vi "Autofocus.vi"(0 "controller in":refnum<k24>, 1 "AbortAutoFocus":bool, 2 "ImageIn":T2, 5 "SafeMaxZ":dbl=86.0 format="%#_13g", 7 "InitialStepSize":dbl=0.1, 9 "Tolerance":dbl=0.005 format="%#_13g", 11 "error in (no error)":errorcluster, 12 "SessionIn":T1) -> (4 "controller out":refnum<k24>, 6 "Image":T2(plugin-control), 8 "N_iterations":dbl, 10 "BestZvalue":dbl, 14 "Session Out":T1, 15 "error out":errorcluster)   [LabVIEW 2021, in "Test VIs.lvclass"]
uses:
  Test VIs/Test VIs.lvclass
  C:/Program Files (x86)/Aerotech/A3200/LabVIEW/2010/Bin/Aerotech.A3200.dll
  Program Files (x86)/Aerotech/A3200/LabVIEW/2010/Bin/Aerotech.A3200.dll
  <vilib>/vision/Image Controls.llb/IMAQ Image.ctl
  <vilib>/userdefined/High Color/IMAQdx.ctl
  <vilib>/Utility/error.llb/DialogType.ctl
  <vilib>/vision/NI_Vision_Development_Module.lvlib
  Drivers/Aerotech A3200/Aerotech.lvlib
  <vilib>/vision/driver/NI_Vision_Acquisition_Software.lvlib
  Classes/Controller/Motion/A3200/A3200.lvclass
panel:
  out "ZvsSD":string
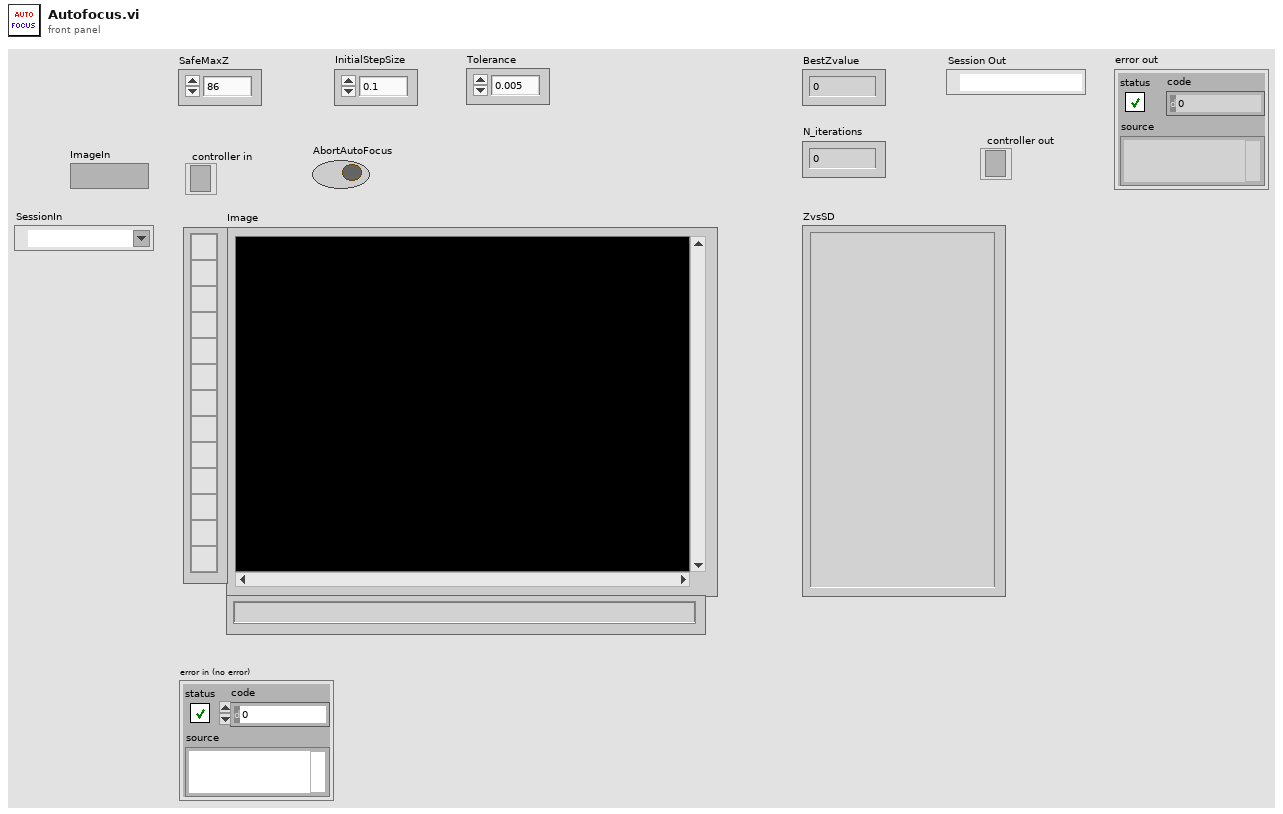
[diagram p1: front panel]
types:
  T1 = typedef "IMAQdx.ctl" = refnum<k21>
  T2 = typedef "IMAQ Image.ctl" = refnum<image>
  T3 = enum32{"Differentiation", "Gradient", "Prewitt", "Roberts", "Sigma", "Sobel"}
  T4 = typedef "Image Type" = u32
  T5 = typedef "DialogType.ctl" = u16
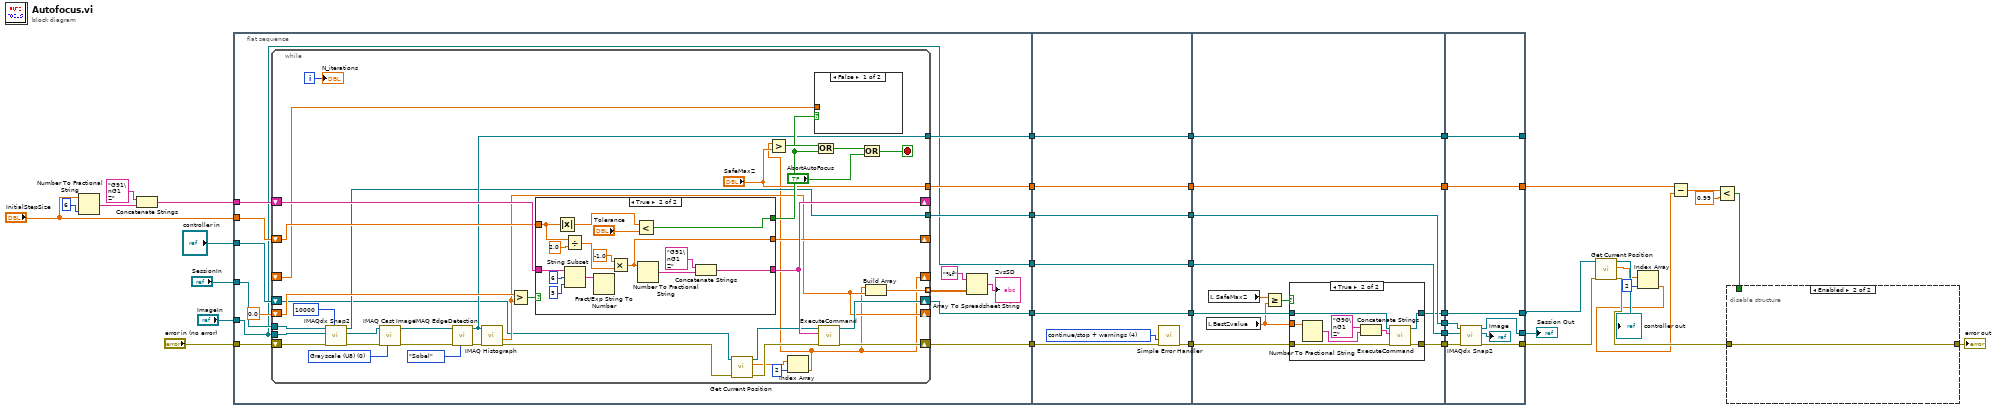
[diagram p0: block diagram]
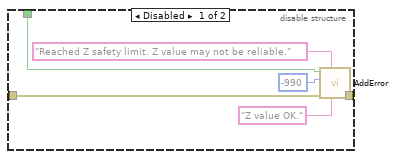
[diagram p2: hidden frame]
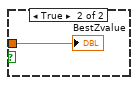
[diagram p3: hidden frame]
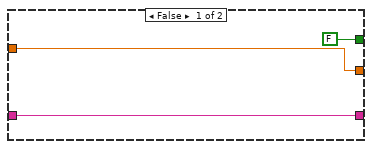
[diagram p4: hidden frame]
diagram:
  n1 = Number To Fractional String(number="InitialStepSize", precision (6)=i16 6) -> (F-format string=w36:string)  [unwired: 2 in]
  n2 = Concatenate Strings("G91\nG1 Z", w36) -> (w38:string)
  n3 = flat-sequence {
    tunnel: "controller in" -> [w55]
    tunnel: "InitialStepSize" -> [w53]
    tunnel: w38 -> [w52]
    tunnel: "error in (no error)" -> [w51]
    tunnel: [w50] -> w23
    tunnel: [w49] -> w21
    tunnel: [w48] -> w19
    tunnel: [w47] -> w17
    tunnel: [w45] -> w15
    tunnel: "SessionIn" -> [w46]
    tunnel: "ImageIn" -> [w44]
    tunnel: [w44] -> w13
    tunnel: w23 -> [w120]
    tunnel: [w120] -> w22
    tunnel: w21 -> [w119]
    tunnel: [w119] -> w20
    tunnel: w19 -> [w114]
    tunnel: [w113] -> w18
    tunnel: w17 -> [w118]
    tunnel: [w118] -> w16
    tunnel: w15 -> [w117]
    tunnel: [w117] -> w14
    tunnel: w13 -> [w116]
    tunnel: [w116] -> w12
    tunnel: w22 -> [w127]
    tunnel: [w124] -> w29
    tunnel: w20 -> [w131]
    tunnel: [w131] -> w28
    tunnel: w18 -> [w126]
    tunnel: [w125] -> w27
    tunnel: w16 -> [w130]
    tunnel: [w130] -> w26
    tunnel: w14 -> [w129]
    tunnel: [w129] -> w25
    tunnel: w12 -> [w128]
    tunnel: [w128] -> w24
    tunnel: [w148] -> _
    tunnel: [w149] -> w31
    tunnel: w29 -> [w150]
    tunnel: w28 -> [w149]
    tunnel: w27 -> [w147]
    tunnel: w26 -> [w148]
    tunnel: [w146] -> w5
    tunnel: [w145] -> w8
    tunnel: w25 -> [w143]
    tunnel: w24 -> [w142]
    tunnel: [w150] -> w7
    frame #0 {
      n4 = while {
        shift-right: [w88] -> w50
        shift-left: w55 -> [w62]
        shift-right: [w89] -> w48
        shift-left: w51 -> [w72]
        shift-right: [w85] -> _
        shift-left: w52 -> [w84]
        shift-right: [w64] -> _
        shift-left: 0.0 -> [w87]
        shift-right: [w81] -> _
        shift-left: w53 -> [w80]
        shift-right: [w56] -> _
        shift-left: _ -> [w79]
        tunnel: ["SafeMaxZ"] -> w49
        tunnel: [w74] -> w47
        tunnel: w44 -> [w70]
        tunnel: w46 -> [w71]
        tunnel: [w68] -> w45
        tunnel: [w65] -> w41 mode=indexing
        i -> [w76]
        stop <- w91 stop-if-true
        w77 = T4 0 items=["Grayscale (U8)", "Grayscale (I16)", "Grayscale (SGL)", "Complex (CSG)", "RGB (U32)", "HSL (U32)", "RGB (U64)", "Grayscale (U16)"] ("Image Type")
        n5 = call <vilib>:"IMAQdx Snap2.vi"("Timeout (ms)"=10000, "error in"=w72, "Image In"=w70, "Session In"=w71) -> ("error out"=w73:errorcluster, "Image Out"=w69:T2, "Session Out"=w68:T1)  [unwired: 5 in]
        n6 = call "IMAQ Cast Image"("Image Type"=w77, "error in (no error)"=w73, "Image Src"=w69) -> ("error out"=w66:errorcluster, "Image Dst Out"=w90:T2)  [unwired: 7 in]
        n7 = call "IMAQ EdgeDetection"("Method"=T3."Sobel", "error in (no error)"=w66, "Image Src"=w90) -> ("error out"=w93:errorcluster, "Image Dst Out"=w74:T2)  [unwired: 7 in]
        n8 = call "IMAQ Histograph"("error in (no error)"=w93, "Image"=w74) -> ("error out"=w60:errorcluster, "Standard  Deviation"=w64:sgl)  [unwired: 6 in, 2 out]
        n9 = Greater?(x=w87, y=w64) -> (0:w86:bool)
        n10 = case shown="True" w86 {
          tunnel: [w97 w111] -> w85
          tunnel: w84 -> [w97 w105]
          tunnel: [FALSE w106] -> w78
          tunnel: [w95 w101] -> w81
          tunnel: w80 -> [w95 w98]
          frame False {
          }
          frame True {
            n11 = Absolute Value(x=w98) -> (abs(x)=w99:dbl)
            n12 = Divide(x=w98, y=2.0) -> (x/y=w100:dbl)
            n13 = String Subset(string=w105, offset (0)=6, length (rest)=5) -> (substring=w102:string)
            n14 = Fract/Exp String To Number(string=w102) -> ()  [unwired: 3 in, 2 out]
            n15 = Multiply(x=-1.0, y=w100) -> (x*y=w101:dbl)
            n16 = Less?(x=w99, y="Tolerance") -> (x < y?=w106:bool)
            n17 = Number To Fractional String(number=w101) -> (F-format string=w110:string)  [unwired: 3 in]
            n18 = Concatenate Strings("G91\nG1 Z", w110) -> (w111:string)
          }
        }
        n19 = call "Get Current Position.vi"("error in (no error)"=w60, "Gantry In"=w62) -> ("error out"=w59:errorcluster, "XYZTheta Out"=w58:dbl[], "Gantry Out"=w61:refnum<k24>)  [unwired: 7 in]
        n20 = Index Array(array=w58, index=2) -> (element=w56:dbl)
        n21 = Greater?(x=w56, y="SafeMaxZ") -> (0:w83:bool)
        n22 = case shown="False" w78 {
          tunnel: w79 -> [_ w94]
          frame False {
          }
          frame True {
            "BestZvalue" <- w94
          }
        }
        n23 = Or(x=w83, y=w78) -> (x .or. y?=w82:bool)
        n24 = call "ExecuteCommand.vi"("error in (no error)"=w59, "Command Code"=w85, "controller in"=w61) -> ("error out"=w89:errorcluster, "controller out"=w88:refnum<k24>)  [unwired: 6 in, 1 out]
        n25 = Or(x=w82, y="AbortAutoFocus") -> (x .or. y?=w91:bool)
        n26 = Build Array(w56, w64) -> (w65:dbl[])
        "N_iterations" <- w76
      }
      n27 = Array To Spreadsheet String(array=w41, 3:"%f" ("format string")) -> (spreadsheet string=→"ZvsSD":string)  [unwired: 1 in]
    }
    frame #1 {
      w115 = T5 4 items=["no dialog", "OK message", "continue or stop message", "OK message + warnings", "continue/stop + warnings"] ("type of dialog (OK msg:1)")
      n28 = call <vilib>:"Simple Error Handler.vi"("type of dialog (OK msg:1)"=w115, "error in (no error)"=w114) -> ("error out"=w113:errorcluster)  [unwired: 3 in, 4 out]
    }
    frame #2 {
      n29 = local read "BestZvalue"() -> (w122:dbl)
      n30 = local read "SafeMaxZ"() -> (w123:dbl)
      n31 = Greater Or Equal?(x=w123, y=w122) -> (x >= y?=w121:bool)
      n32 = case shown="True" w121 {
        tunnel: w127 -> [w133 w141]
        tunnel: w126 -> [w132 w140]
        tunnel: [w132 w136] -> w125
        tunnel: [w133 w135] -> w124
        tunnel: w122 -> [_ w134]
        frame False {
        }
        frame True {
          n33 = Number To Fractional String(number=w134) -> (F-format string=w139:string)  [unwired: 3 in]
          n34 = Concatenate Strings("G90\nG1 Z", w139) -> (w137:string)
          n35 = call "ExecuteCommand.vi"("error in (no error)"=w140, "Command Code"=w137, "controller in"=w141) -> ("error out"=w136:errorcluster, "controller out"=w135:refnum<k24>)  [unwired: 6 in, 1 out]
        }
      }
    }
    frame #3 {
      n36 = call <vilib>:"IMAQdx Snap2.vi"("error in"=w147, "Image In"=w142, "Session In"=w143) -> ("error out"=w146:errorcluster, "Image Out"=→"Image":T2, "Session Out"=w145:T1)  [unwired: 6 in]
    }
  }
  n37 = call "Get Current Position.vi"("error in (no error)"=w5, "Gantry In"=w7) -> ("error out"=w4:errorcluster, "XYZTheta Out"=w3:dbl[], "Gantry Out"=→"controller out":refnum<k24>)  [unwired: 7 in]
  n38 = Index Array(array=w3, index=2) -> (element=w2:dbl)
  n39 = Subtract(x=w31, y=w2) -> (x-y=w35:dbl)
  n40 = Less?(x=w35, y=0.99) -> (x < y?=w33:bool)
  n41 = disable-structure shown="Enabled" {
    disable-tunnel: w33 -> [w156 _]
    disable-tunnel: [w154 w157] -> w32
    disable-tunnel: w4 -> [w151 w157]
    frame Disabled {
      n42 = call "AddError.vi"("NoErrorMessage"="Z value OK.", "ErrorMessage"="Reached Z safety limit. Z value may not be reliable.", "error in"=w151, "code"=-990, "Error?"=w156) -> ("Error out"=w154:errorcluster)  [unwired: 6 in]
    }
    frame Enabled {
    }
  }
  "error out" <- w32
  "Session Out" <- w8
